vi "Rx Begin.vi"(8 "error in (no error)":errorcluster, 11 "Transfer Group in":refnum<class "Transfer Group.lvclass">) -> (0 "error out":errorcluster, 3 "Transfer Group out":refnum<class "Transfer Group.lvclass">)   [LabVIEW 2019, in "DSF Core.lvlib" / "Transfer Group.lvclass"]
uses:
  Transfer Group.lvclass
  Transfer Group.lvclass/Transfer Group.ctl
  Performance/Performance.lvclass/Performance.ctl
  Performance/Performance.lvclass
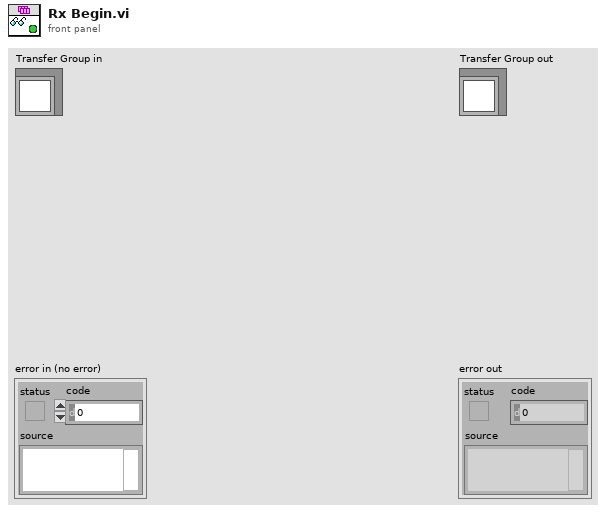
[diagram p1: front panel]
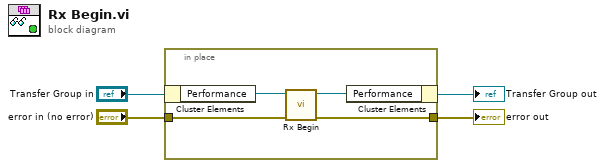
[diagram p0: block diagram]
diagram:
  n1 = in-place {
    in-place-border: "error in (no error)" -> [w6]
    in-place-border: [w7] -> w2
    n2 = in-place-cluster #1("Transfer Group in") -> ("Performance"=w5:refnum<class "Performance.lvclass">)
    n3 = call "Rx Begin.vi"("error in (no error)"=w6, "Performance in"=w5) -> ("error out"=w7:errorcluster, "Performance out"=w8:refnum<class "Performance.lvclass">)  [unwired: 8 in]
    n4 = in-place-cluster #1("Performance"=w8) -> (→"Transfer Group out":refnum<class "Transfer Group.lvclass">)
  }
  "error out" <- w2
